vi "TurnAMP_ON_OFF.vi"() -> ()   [LabVIEW 2019]
uses:
  <vilib>/Platform/TimedLoop/XDataNode/timing_clust.ctl
  <vilib>/Platform/TimedLoop/XDataNode/nitl_modes.ctl
  <vilib>/Platform/TimedLoop/XDataNode/wakeup.ctl
  <vilib>/FPGAPlugInAG/myRIO-1900/niLvFpga_Open_myRIO-1900.vi
  <vilib>/rvi/interface/common/dynamic/niFpgaDynamicAddResources.vi
  <vilib>/Utility/error.llb/Error Cluster From Error Code.vi
  <vilib>/rvi/errors/niLvFpgaAdjustHostInterfaceError.vi
  <vilib>/platform/TimedLoop/XDataNode/XDataNode.xnode
  <vilib>/rvi/interface/nirviOpenFPGA/nirviOpenFPGA.xnode
  FPGA Bitfiles/studentchallenge_FPGATarget_FPGA1RADC1WDAC2A_R8uuw9uWLNg.lvbitx
  <vilib>/rvi/interface/nirviReadWriteControl/nirviReadWriteControl.xnode
  <vilib>/Platform/TimedLoop/XDataNode/XDNodeRunTimeDep.lvlib
  NiFpgaLv.dll
  <vilib>/rvi/interface/Simulation/niFpgaSimulationCallBeginRW.vi
panel:
  in  "Manual airbearing coil (V)":dbl format="%#_3f"
  out "Finished Late? [i-1]":bool
  out "Capacitance gage (um)":dbl=-0.020783679448250613 format="%#_5f"
  in  "?":bool
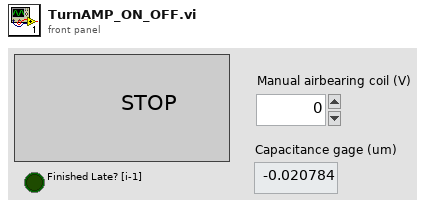
[diagram p1: front panel]
types:
  T1 = typedef "XDNodeRunTimeDep.lvlib/timing_clust.ctl" = cluster{"Expected End [f-1]":u64, "Actual End [f-1]":u64, "Finished Late? [f-1]":bool, "Expected End [i-1]":u64, "Actual End [i-1]":u64, "Finished Late? [i-1]":bool, "Expected Start [i]":u64, "Actual Start [i]":u64, "Expected Start [f]":u64, "Actual Start [f]":u64, "Source Name":string, "Structure Name":string, "Period":i64, "Deadline":i64, "Offset":i64, "Start":i64, "Priority":i32, "Timeout":i32, "Mode":T2, "Wakeup Reason":T3, "Error":errorcluster, "Source Type":string, "Secondary Source Type":string, "Global End Time":u64, "Global Start Time":u64, "Frame Duration":u64, "Iteration Duration":u64, "Assigned CPU":i32, "I/O Scan Engine Mode":u32}
  T2 = typedef "XDNodeRunTimeDep.lvlib/nitl_modes.ctl" = enum32{"No Change", "Process missed periods, maintain original phase", "Discard missed periods, maintain original phase", "Process missed periods, ignore original phase", "Discard missed periods, ignore original phase"}
  T3 = typedef "XDNodeRunTimeDep.lvlib/wakeup.ctl" = enum32{"Normal", "Aborted", "Asynchronous wakeup", "Timing source error", "Timed loop error", "Timeout"}
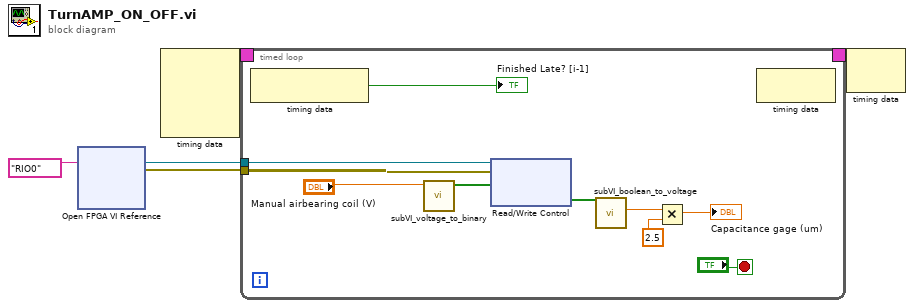
[diagram p0: block diagram]
diagram:
  n1 = xnode "Open FPGA VI Reference"("resource name"=tag "RIO0") -> ("FPGA VI Reference Out"=w2:refnum<k20>, "error out"=w1:errorcluster)  [unwired: 1 in]
  n2 = node-c288() -> (w5:T1)  [unwired: 4 in]
  n3 = timed-loop {
    tunnel: w2 -> [w14]
    tunnel: w1 -> [w13]
    timing: w5 -> [_]
    timing-out: [_] -> w4
    stop <- "?" stop-if-true
    n4 = node-c288() -> (→"Finished Late? [i-1]":bool)  [unwired: 1 in]
    n5 = call "subVI_voltage_to_binary.vi"("voltage"="Manual airbearing coil (V)") -> ("binary"=w9:bool[])  [unwired: 10 in]
    n6 = xnode "Read/Write Control"("FPGA VI Reference In"=w14, "error in"=w13, "DAC 1 write"=w9) -> ("ADC Read"=w6:bool[])  [unwired: 2 out]
    n7 = call "subVI_boolean_to_voltage.vi"("ADC read"=w6) -> ("V"=w7:dbl)  [unwired: 10 in]
    n8 = Multiply(x=w7, y=2.5) -> (x*y=→"Capacitance gage (um)":dbl)
    n9 = node-c288() -> ()  [unwired: 1 in, 1 out]
  }
  n10 = node-c288(w4) -> ()  [unwired: 1 out]
